vi "Calc Tuning Params.vi"(4 "tuning parameters\n(0:auto-calc)":T1 {"peak threshold" min=0.0 format="%.2f"; "max noise" min=0.0 format="%.2f"}, 5 "Y data":dbl[](array[numeric]) format="%.2f") -> (0 "min points to fit":i32, 1 "max noise":dbl format="%.2f", 2 "peak threshold":dbl format="%.2f")   [LabVIEW 2012]
doc: "When a parameter used for peak detection and baseline determination is zero, this VI calculates its value from the Y data. Non-zero values are left unchanged. Do not use zero values unless the Y array contains all the data (post-processing), otherwise the values cannot be calculated correctly.\n\nUse the help window to read the descriptions of the individual controls for more information about this VI's inputs and outputs."
uses:
  Tuning.ctl
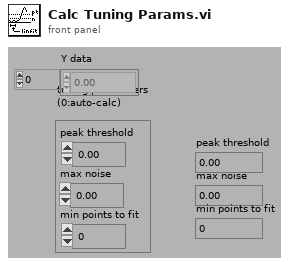
[diagram p1: front panel]
types:
  T1 = typedef "Tuning.ctl" = cluster{"max noise":dbl, "min points to fit":i32, "peak threshold":dbl}
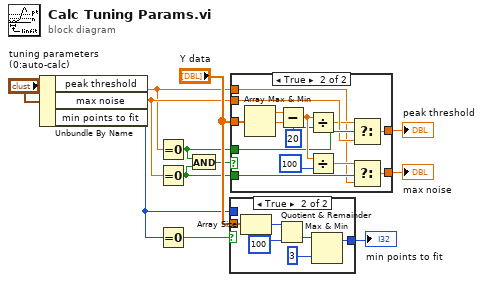
[diagram p0: block diagram]
diagram:
  n1 = Unbundle By Name("tuning parameters\n(0:auto-calc)") -> ("peak threshold"=w6:dbl, "max noise"=w7:dbl, "min points to fit"=w5:i32)
  n2 = Equal To 0?(x=w6) -> (x = 0?=w3:bool)
  n3 = Equal To 0?(x=w7) -> (x = 0?=w2:bool)
  n4 = Equal To 0?(x=w5) -> (x = 0?=w11:bool)
  n5 = And(x=w3, y=w2) -> (x .and. y?=w9:bool)
  n6 = case shown="True" w11 {
    tunnel: [w13 w14] -> w8
    tunnel: "Y data" -> [_ w16]
    tunnel: w5 -> [w13 _]
    frame False {
    }
    frame True {
      n7 = Array Size(array=w16) -> (size(s)=w18:i32)
      n8 = Quotient & Remainder(x=w18, y=100) -> (floor(x/y)=w17:i32)  [unwired: 1 out]
      n9 = Max & Min(x=w17, y=3) -> (max(x,y)=w14:i32)  [unwired: 1 out]
    }
  }
  "min points to fit" <- w8
  n10 = case shown="True" w9 {
    tunnel: [w21 w22] -> w1
    tunnel: [w20 w28] -> w4
    tunnel: "Y data" -> [_ w30]
    tunnel: w7 -> [w21 w27]
    tunnel: w6 -> [w20 w23]
    tunnel: w3 -> [_ w29]
    tunnel: w2 -> [_ w24]
    frame False {
    }
    frame True {
      n11 = Array Max & Min(array=w30) -> (max value=w35:dbl, min value=w34:dbl)  [unwired: 2 out]
      n12 = Subtract(x=w35, y=w34) -> (x-y=w33:dbl)
      n13 = Divide(x=w33, y=20) -> (x/y=w26:dbl)
      n14 = Divide(x=w33, y=100) -> (x/y=w25:dbl)
      n15 = Select(t=w26, s=w29, f=w27) -> (s? t:f=w28:dbl)
      n16 = Select(t=w25, s=w24, f=w23) -> (s? t:f=w22:dbl)
    }
  }
  "max noise" <- w1
  "peak threshold" <- w4
